vi "GetLongFilePath.vi"(0 "path":path=path "C:/Data/Junk", 1 "replace \\ by \\\\":bool, 7 "file name":string="tst", 9 "X Row":i32, 11 "Y Row":i32, 12 "Optical Input":i32, 13 "Optical Output":i32, 14 "Scan":i32) -> (6 "final path":string, 10 "complete path":path=path "C:/Data/Junk")   [LabVIEW 2011]
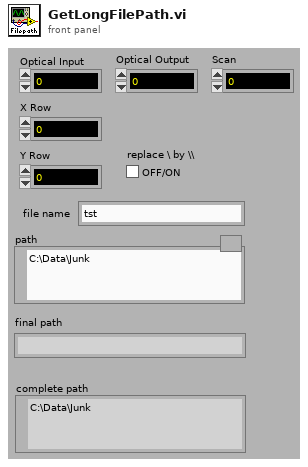
[diagram p1: front panel]
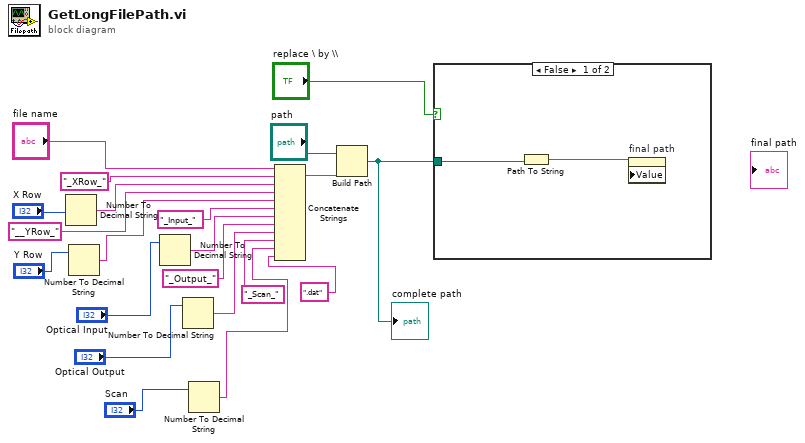
[diagram p0: block diagram]
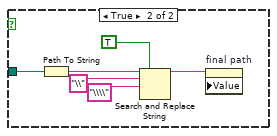
[diagram p2: hidden frame]
diagram:
  n1 = Number To Decimal String(number="X Row") -> (decimal integer string=w18:string)  [unwired: 1 in]
  n2 = Number To Decimal String(number="Y Row") -> (decimal integer string=w13:string)  [unwired: 1 in]
  n3 = Number To Decimal String(number="Optical Input") -> (decimal integer string=w7:string)  [unwired: 1 in]
  n4 = Number To Decimal String(number="Optical Output") -> (decimal integer string=w5:string)  [unwired: 1 in]
  n5 = Number To Decimal String(number="Scan") -> (decimal integer string=w2:string)  [unwired: 1 in]
  n6 = Concatenate Strings("file name", "_XRow_", w18, "__YRow_", w13, "_Input_", w7, "_Output_", w5, "_Scan_", w2, ".dat") -> (w17:string)
  n7 = Build Path(base path="path", name or relative path=w17) -> (appended path=w14:path)
  "complete path" <- w14
  n8 = case shown="False" "replace \\ by \\\\" {
    tunnel: w14 -> [w23 w25]
    frame False {
      n9 = Path To String(path=w23) -> (string=w22:string)
      n10 = property on="final path" class="Str"("Value"=w22) -> ()  [unwired: 2 in, 2 out]
    }
    frame True {
      n11 = Path To String(path=w25) -> (string=w26:string)
      n12 = Search and Replace String(replace all?=TRUE, input string=w26, search string="\\", replace string="\\\\") -> (result string=w24:string)  [unwired: 4 in, 3 out]
      n13 = property on="final path" class="Str"("Value"=w24) -> ()  [unwired: 2 in, 2 out]
    }
  }
